vi "ArmAbsolutePoseToXYPoint.vi"(1 "ArmAbsolutePose":T2) -> (0 "2DPoint":T1)   [LabVIEW 2018]
uses:
  TypeDefs/ArmAbsolutePosition.ctl
  ArgosLib/Path Planning/TypeDefs/Point2D.ctl
  ArgosLib/ArgosLib.lvlib
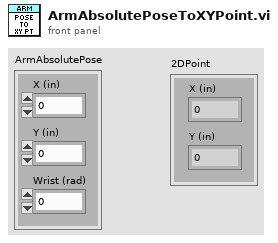
[diagram p1: front panel]
types:
  T1 = typedef "ArgosLib.lvlib/Point2D.ctl" = cluster{"X (in)":dbl, "Y (in)":dbl}
  T2 = typedef "ArmAbsolutePosition.ctl" = cluster{"X (in)":dbl, "Y (in)":dbl, "Wrist (rad)":dbl}
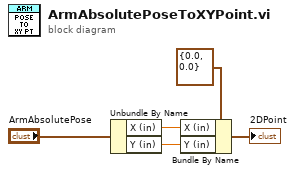
[diagram p0: block diagram]
diagram:
  n1 = Unbundle By Name("ArmAbsolutePose") -> ("X (in)"=w2:dbl, "Y (in)"=w1:dbl)
  n2 = Bundle By Name(cluster=T1 {"X (in)"=0.0, "Y (in)"=0.0} ("2DPoint"), "X (in)"=w2, "Y (in)"=w1) -> (→"2DPoint":T1)
